vi "Migrate all Measurement Dependencies.vi"(0 "Project path":path, 1 "Measurement paths":path[](array[path]), 2 "Init":T1[](array[typedef]), 5 "Plug-in names":string[](array[string]), 7 "Measurement dependencies":path[][](array[path]), 9 "Outside items":string[](array[string]), 11 "error in (no error)":errorcluster, 12 "Shared dependent VIs":path[](array[path])) -> (6 "DestinationDirectory":path[](array[path]), 15 "error out":errorcluster)   [LabVIEW 2021, in "Multiple Migrator.lvlib"]
uses:
  Multiple Migrator.lvlib
  controls/Library Info.ctl
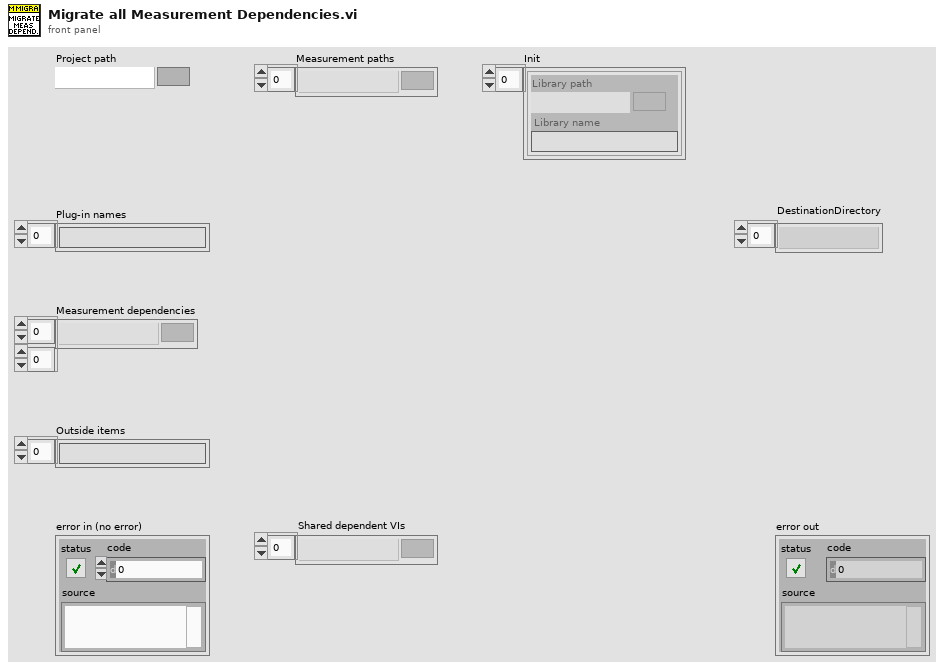
[diagram p1: front panel]
types:
  T1 = typedef "Multiple Migrator.lvlib/Library Info.ctl" = cluster{"Library path":path, "Library name":string}
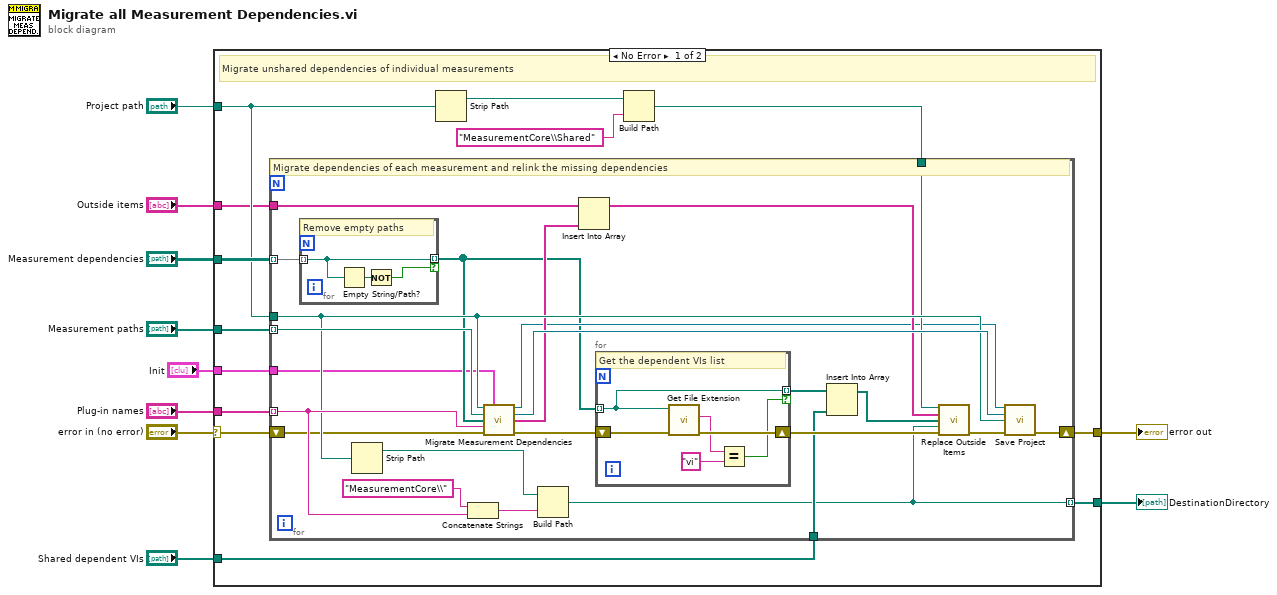
[diagram p0: block diagram]
diagram:
  n1 = case shown="No Error" "error in (no error)" {
    selector: "error in (no error)" -> [w22 w57]
    tunnel: "Measurement dependencies" -> [w23 _]
    tunnel: "Project path" -> [w18 _]
    tunnel: "Outside items" -> [w17 _]
    tunnel: "Measurement paths" -> [w16 _]
    tunnel: "Plug-in names" -> [w15 _]
    tunnel: [w14 w57] -> w4
    tunnel: "Shared dependent VIs" -> [w13 _]
    tunnel: [w12 _] -> w2
    tunnel: "Init" -> [w11 _]
    frame No Error {
      # "Migrate unshared dependencies of individual measurements"
      n2 = Strip Path(path=w18) -> (stripped path=w19:path)  [unwired: 1 out]
      n3 = Build Path(base path=w19, name or relative path="MeasurementCore\\Shared" ("string")) -> (appended path=w21:path)
      n4 = for {
        tunnel: w18 -> [w39]
        tunnel: w16 -> [w44] mode=indexing
        tunnel: w15 -> [w41] mode=indexing
        tunnel: w17 -> [w38]
        tunnel: w21 -> [w35]
        shift-right: [w45] -> w14
        shift-left: w22 -> [w33]
        tunnel: w23 -> [w32] mode=indexing
        tunnel: w13 -> [w27]
        tunnel: [w25] -> w12 mode=indexing
        tunnel: w11 -> [w24]
        # "Migrate dependencies of each measurement and relink the missing dependencies"
        n5 = for {
          tunnel: w32 -> [w55] mode=indexing
          tunnel: [w55] -> w29 mode=indexing if=w54
          # "Remove empty paths"
          n6 = Empty String/Path?(string/path=w55) -> (empty?=w56:bool)
          n7 = Not(x=w56) -> (.not. x?=w54:bool)
        }
        n8 = Strip Path(path=w39) -> (stripped path=w40:path)  [unwired: 1 out]
        n9 = Concatenate Strings("MeasurementCore\\" ("string"), w41) -> (w30:string)
        n10 = call "Migrate Measurement Dependencies.vi"("Project path"=w39, "Init"=w24, "Measurement path"=w44, "Dependencies path"=w29, "Plug-in name"=w41, "error in (no error)"=w33) -> ("Project reference"=w34:refnum<vi>, "MeasurementCore reference"=w43:refnum<vi>, "Outside items"=w37:string[], "error out"=w47:errorcluster)  [unwired: 6 in]
        n11 = Build Path(base path=w40, name or relative path=w30) -> (appended path=w25:path)
        n12 = Insert Into Array(array=w38, new element=w37) -> (w36:string[])  [unwired: 1 in]
        n13 = for {
          shift-right: [w52] -> w31
          shift-left: w47 -> [w53]
          tunnel: w29 -> [w51] mode=indexing
          tunnel: [w51] -> w28 mode=indexing if=w48
          # "Get the dependent VIs list"
          n14 = call <vilib>:"Get File Extension.vi"("error in (no error)"=w53, "file"=w51) -> ("error out"=w52:errorcluster, "lowercase file extension"=w49:string)  [unwired: 5 in, 3 out]
          n15 = Equal?(x=w49, y="vi" ("x")) -> (x = y?=w48:bool)
        }
        n16 = Insert Into Array(array=w28, new element=w27) -> (w26:path[])  [unwired: 1 in]
        n17 = call "Replace Outside Items.vi"("Shared directory"=w35, "OutsideVIs"=w36, "Dependent VIs"=w26, "Measurement directory"=w25, "error in (no error)"=w31) -> ("error out"=w46:errorcluster)  [unwired: 10 in]
        n18 = call "Save Project.vi"("Project reference"=w34, "MeasurementCore reference"=w43, "Project path"=w39, "error in (no error)"=w46) -> ("error out"=w45:errorcluster)  [unwired: 11 in]
      }
    }
    frame Error {
      # "Pass"
    }
  }
  "error out" <- w4
  "DestinationDirectory" <- w2
